vi "Set Dt.vi"(8 "error in (no error)":errorcluster, 10 "Dt":dbl, 11 "Fit Exponential in":refnum<class "Fit Exponential.lvclass">) -> (0 "error out":errorcluster, 3 "Fit Exponential out":refnum<class "Fit Exponential.lvclass">)   [LabVIEW 2016, in "Exponential Fit Library.lvlib" / "Fit Exponential.lvclass"]
uses:
  Fit Exponential.lvclass
  Fit Exponential.lvclass/Fit Exponential.ctl
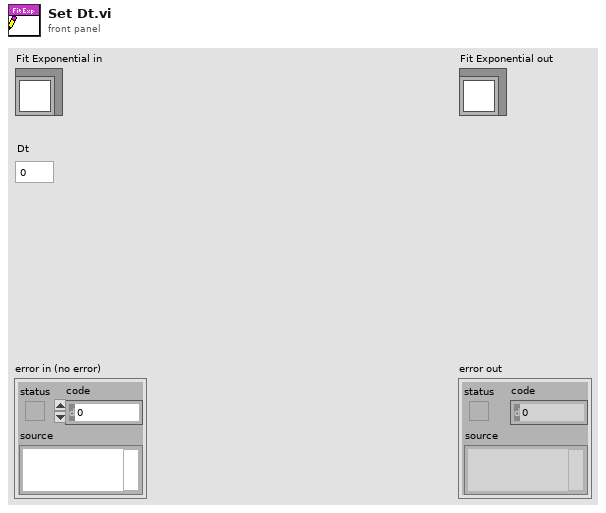
[diagram p1: front panel]
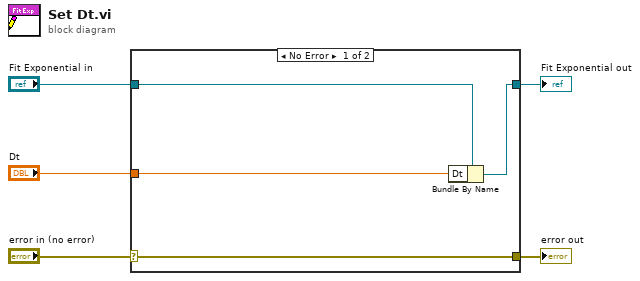
[diagram p0: block diagram]
diagram:
  n1 = case shown="No Error" "error in (no error)" {
    selector: "error in (no error)" -> [w9 w10]
    tunnel: [w9 w10] -> w4
    tunnel: [w7 w11] -> w2
    tunnel: "Fit Exponential in" -> [w8 w11]
    tunnel: "Dt" -> [w6 _]
    frame No Error {
      n2 = Bundle By Name(cluster=w8, "Dt"=w6) -> (w7:refnum<class "Fit Exponential.lvclass">)
    }
    frame Error {
    }
  }
  "error out" <- w4
  "Fit Exponential out" <- w2
